vi "m_globals.vi"() -> ()   [LabVIEW 2017]
panel:
  in  "usb comd resp timeout":i32=30000
  out "usbhandle":i32=1
  in  "sFileName":string="\\\\.\\EzUsb-0"
  out "bndslitsselectorkey":string="bndslitsselector"
  out "BndSlits":bool
  in  "send command delay":i32=20
  out "INI file name":string="cs130.ini"
  out "fltrautokey":string="fltrauto"
  out "gratautokey":string="gratauto"
  out "fltrposkey":string="fltrpos"
  out "fltrwavekey":string="fltrwave"
  out "gratposkey":string="gratpos"
  out "gratwavekey":string="gratwave"
  in  "Fltr Wave Table":dbl[](array[numeric])=[inf, inf, inf, inf, inf, inf, inf, inf] format="%.2f"
  out "Fltr Table On":bool
  in  "Fltr position table":u16[](array[numeric])=[1, 1, 1, 1, 1, 1, 1, 1] min=1 max=6 step=1
  in  "Grat Wave Table":dbl[](array[numeric])=[inf, inf] format="%.2f"
  out "Grat Table On":bool
  in  "grat position table":u16[](array[numeric])=[1, 1] min=1 max=6 step=1
  out "gpibbuskey":string="gpibbus"
  out "INI":path=path "c:/windows/cs130.ini"
  out "gpibaddresskey":string="gpibaddress"
  out "section":string="Cornerstone130"
  in  "wavelength":dbl format="%.2f"
  in  "terminator":i16=10 min=0 max=30
  in  "gpib_timeout":i32=1000
  in  "MAXLEN":i32=61 min=0 max=30
  in  "mode":i16 min=0 max=30
  in  "bus":i32 min=0 max=30
  in  "address":i16=4 min=0 max=30
  # "Wave tables are kept in nm"
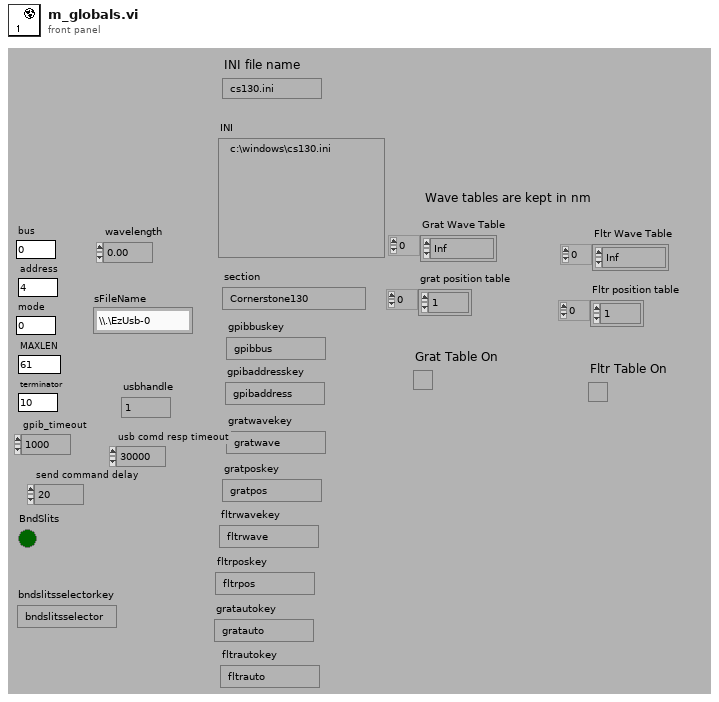
[diagram p1: front panel]
diagram:
